vi "Calculate wave for bits.vi"(0 "No. Of Bits":i32, 5 "SCL DATA IN":u8[](array[numeric]), 7 "SCL Transitions In":u32[](array[numeric]), 9 "SDA Transitions In":u32[](array[numeric]), 11 "Time Params":T1={"f_SCL(KHz)"=100, "t_HIGH (ns)"=5000, "t_LOW (ns)"=5000, "t_SU;STA (ns)"=4700, "t_HD;STA (ns)"=4000, "t_SU;DAT (ns)"=2500, "t_HD;DAT (ns)"=2500, "t_SU;STO (ns)"=4000, "t_BUF (ns)"=4700} {"t_HIGH (ns)" max=500000 step=1 format="%#.0f"; "t_LOW (ns)" max=50000 step=1 format="%#.0f"; "f_SCL(KHz)" min=10 max=1000 step=1}) -> (4 "SCL DATA OUT":u8[](array[numeric]), 6 "SCL Transitions Out":u32[](array[numeric]), 8 "SDA Transitions Out":u32[](array[numeric]))   [LabVIEW 2020, in "TX Speed.lvclass"]
uses:
  TX Speed.lvclass
  TypeDef/Timing Parameters Cluster.ctl
  TX Speed.lvclass/TX Speed.ctl
  I2C Controller Lib.lvlib
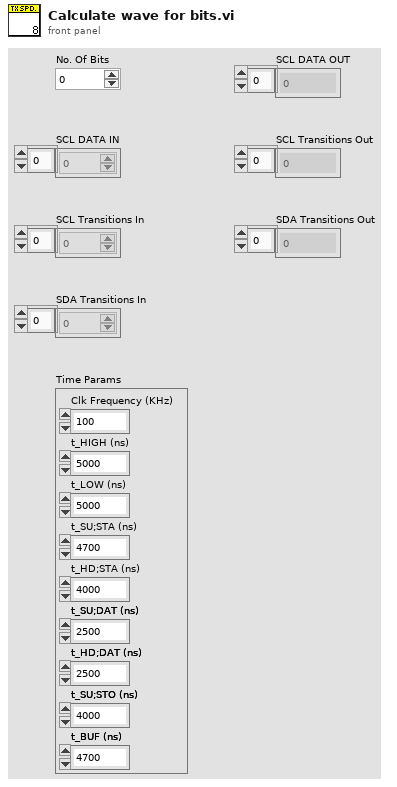
[diagram p1: front panel]
types:
  T1 = typedef "I2C Controller Lib.lvlib/Timing Parameters Cluster.ctl" = cluster{"f_SCL(KHz)":u32, "t_HIGH (ns)":u32, "t_LOW (ns)":u32, "t_SU;STA (ns)":u32, "t_HD;STA (ns)":u32, "t_SU;DAT (ns)":u32, "t_HD;DAT (ns)":u32, "t_SU;STO (ns)":u32, "t_BUF (ns)":u32}
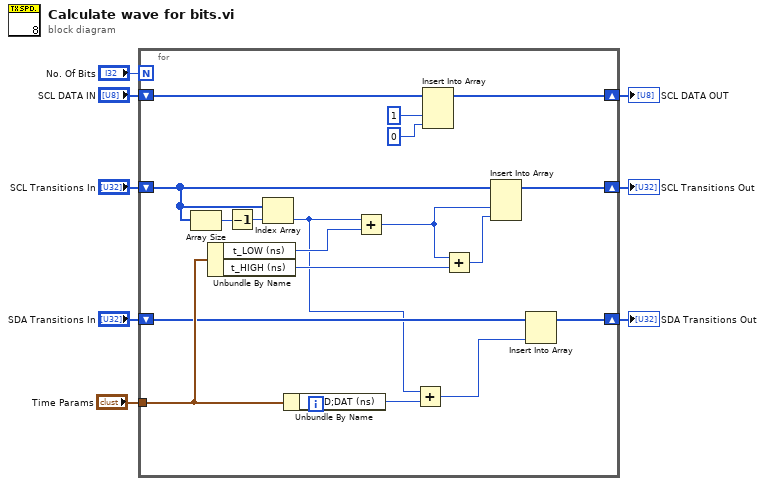
[diagram p0: block diagram]
diagram:
  n1 = for {
    N: "No. Of Bits" -> [_]
    tunnel: "Time Params" -> [w21]
    shift-right: [w14] -> w2
    shift-left: "SDA Transitions In" -> [w11]
    shift-right: [w23] -> w4
    shift-left: "SCL DATA IN" -> [w26]
    shift-right: [w22] -> w3
    shift-left: "SCL Transitions In" -> [w18]
    n2 = Array Size(array=w18) -> (size(s)=w20:i32)
    n3 = Unbundle By Name(w21) -> ("t_LOW (ns)"=w17:u32, "t_HIGH (ns)"=w16:u32)
    n4 = Decrement(x=w20) -> (x-1=w19:i32)
    n5 = Index Array(array=w18, index=w19) -> (element=w9:u32)
    n6 = Unbundle By Name(w21) -> ("t_HD;DAT (ns)"=w13:u32)
    n7 = Add(x=w9, y=w17) -> (x+y=w10:u32)
    n8 = Add(x=w9, y=w13) -> (x+y=w12:u32)
    n9 = Insert Into Array(array=w26, new element #1=u8 1 ("new element/subarray"), new element #2=u8 0 ("new element/subarray")) -> (w23:u8[])  [unwired: 1 in]
    n10 = Add(x=w10, y=w16) -> (x+y=w15:u32)
    n11 = Insert Into Array(array=w18, new element #1=w10, new element #2=w15) -> (w22:u32[])  [unwired: 1 in]
    n12 = Insert Into Array(array=w11, new element=w12) -> (w14:u32[])  [unwired: 1 in]
  }
  "SCL DATA OUT" <- w4
  "SCL Transitions Out" <- w3
  "SDA Transitions Out" <- w2
